vi "UE9 Single AIN Example Loop.vi"() -> ()   [LabVIEW 2021]
panel:
  out "Iteration#":i32
  in  "Interval [ms]":u32=500
  in  "stop":bool
  out "Error Message":string
  in  "Resolution":i32=12
  in  "AIN Range":u16(ring) items=["LJ_rgBIP5V", "LJ_rgUNI5V", "LJ_rgUNI2P5V", "LJ_rgUNI1P25V", "LJ_rgUNIP625V"]
  out "error out":errorcluster
  out "Value Read":dbl format="%.6f"
  in  "Channel #":i32
  # "Aquires 1 analog input channel from the first found UE9 over USB.\n\nThis is the same as \"UE9 Single AIN Example.vi\", but the AIN read is put\nin a loop.  Note that only the AIN read itself is in the loop, not the configuration,\nso the control inputs (channel#, range, resolution) can't be changed after\nyou start running the VI."
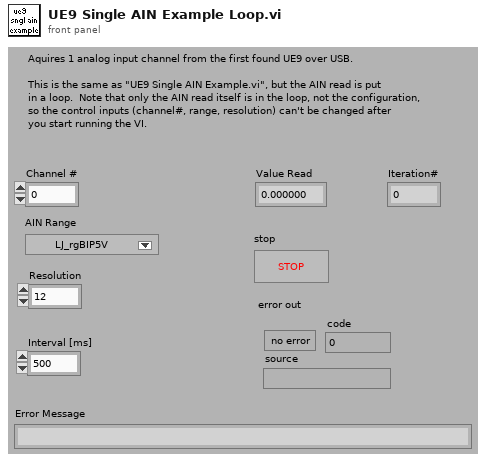
[diagram p1: front panel]
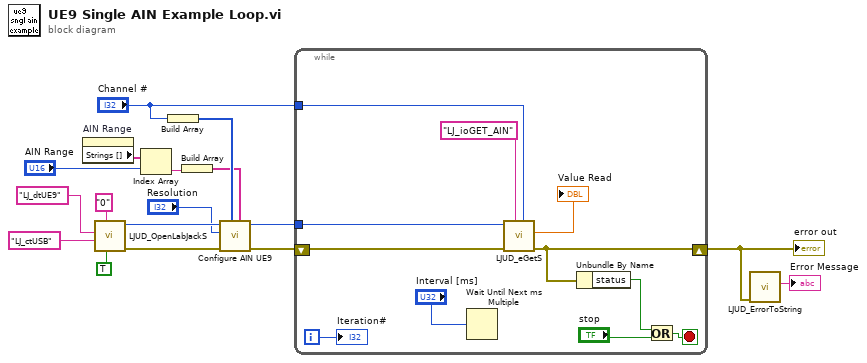
[diagram p0: block diagram]
diagram:
  n1 = property on="AIN Range" class="Ring (strict)"() -> ("Strings []"=w8:string[])  [unwired: 2 in, 2 out]
  n2 = call "LJUD_OpenLabJackS.vi"("FirstFound"=TRUE, "Address"="0", "ConnectionType"="LJ_ctUSB", "DeviceType"="LJ_dtUE9") -> ("error out"=w16:errorcluster, "Handle"=w17:i32)  [unwired: 5 in, 1 out]
  n3 = Index Array(array=w8, index="AIN Range") -> (element=w6:string)
  n4 = Build Array("Channel #") -> (w10:i32[])
  n5 = Build Array(w6) -> (w5:string[])
  n6 = call "Configure AIN UE9.vi"("Ranges"=w5, "Channels"=w10, "error in"=w16, "Resolution"="Resolution", "Handle In"=w17) -> ("error out"=w3:errorcluster, "Handle Out"=w1:i32)  [unwired: 5 in]
  n7 = while {
    tunnel: w1 -> [w22]
    shift-left: w3 -> [w24]
    shift-right: [w23] -> w2
    tunnel: "Channel #" -> [w27]
    i -> [w18]
    stop <- w26 stop-if-true
    n8 = Wait Until Next ms Multiple(millisecond multiple="Interval [ms]") -> ()  [unwired: 1 out]
    n9 = call "LJUD_eGetS.vi"("Channel"=w27, "IOType"="LJ_ioGET_AIN", "error in"=w24, "Handle In"=w22) -> ("error out"=w23:errorcluster, "Value Read"=→"Value Read":dbl)  [unwired: 5 in, 1 out]
    n10 = Unbundle By Name(w23) -> ("status"=w25:bool)
    n11 = Or(x=w25, y="stop") -> (x .or. y?=w26:bool)
    "Iteration#" <- w18
  }
  "error out" <- w2
  n12 = call "LJUD_ErrorToString.vi"("error in"=w2) -> ("String"=→"Error Message":string)  [unwired: 10 in]
